vi "Gyro Calibration.vi"(5 "Port (Port 1)":T2=2 items=["Port 1", "Port 2", "Port 3", "Port 4"], 9 "NXT/EV3":T1) -> (0 "Boolean":bool, 1 "Degrees":sgl, 3 "NXT/EV3":T1)   [LabVIEW 2016]
uses:
  <vilib>/NXT/Block Support/NXT_InputPort.ctl
  <vilib>/NXT/Subs/LVHSConnector.ctl
  <vilib>/NXT/LegoClasses/BrickReference/BrickReference.lvclass
  <vilib>/NXT/Dual Mode Library/Sensors/EV3_Gyro_Angle.vi
  <vilib>/NXT/Dual Mode Library/Sensors/EV3_Gyro_Rate.vi
  <vilib>/NXT/Dual Mode Library/Waits/Wait_Num(msec).vi
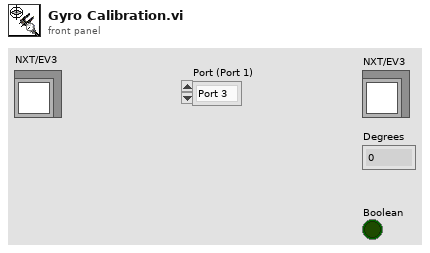
[diagram p1: front panel]
types:
  T1 = typedef "LVHSConnector.ctl" = refnum<class "BrickReference.lvclass">
  T2 = typedef "NXT_InputPort.ctl" = u32
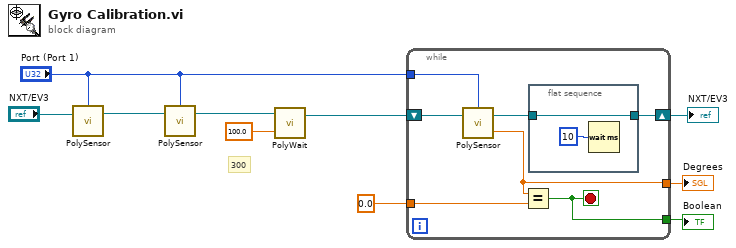
[diagram p0: block diagram]
diagram:
  # "300"
  n1 = call-poly <vilib>:"PolySensor.vi"("NXT/EV3"="NXT/EV3", "Port (Port 1)"="Port (Port 1)") -> ("NXT/EV3"=w8:T1)  [unwired: 1 in, 1 out]
  n2 = call-poly <vilib>:"PolySensor.vi"("NXT/EV3"=w8, "Port (Port 1)"="Port (Port 1)") -> ("NXT/EV3"=w7:T1)  [unwired: 1 in, 1 out]
  n3 = call-poly <vilib>:"PolyWait.vi"("Time (100 msec)"=sgl 100.0 ("Time (1 sec)"), "NXT/EV3"=w7) -> ("NXT/EV3"=w5:T1)  [unwired: 2 in]
  n4 = while {
    shift-right: [w14] -> w9
    shift-left: w5 -> [w16]
    tunnel: "Port (Port 1)" -> [w17]
    tunnel: sgl 0.0 ("Degree (180)") -> [w15]
    tunnel: [w12] -> w3
    tunnel: [w11] -> w2
    stop <- w11 stop-if-true
    n5 = call-poly <vilib>:"PolySensor.vi"("NXT/EV3"=w16, "Port (Port 1)"=w17) -> ("Degrees"=w12:sgl, "NXT/EV3"=w13:T1)  [unwired: 1 in]
    n6 = Equal?(x=w12, y=w15) -> (x = y?=w11:bool)
    n7 = flat-sequence {
      tunnel: w13 -> [w19]
      tunnel: [w19] -> w14
      frame #0 {
        n8 = Wait (ms)(milliseconds to wait=u32 10) -> ()  [unwired: 1 out]
      }
    }
  }
  "NXT/EV3" <- w9
  "Degrees" <- w3
  "Boolean" <- w2
